vi "TempMonitor_VoltageToTemp.vi"(1 "Output Voltage":dbl) -> (0 "Temp (C)":dbl)   [LabVIEW 2012]
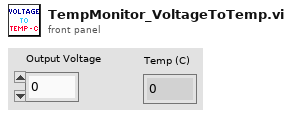
[diagram p1: front panel]
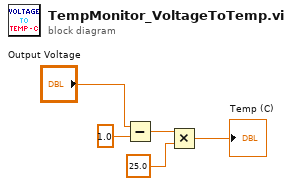
[diagram p0: block diagram]
diagram:
  n1 = Subtract(x="Output Voltage", y=1.0) -> (x-y=w4:dbl)
  n2 = Multiply(x=w4, y=25.0) -> (x*y=→"Temp (C)":dbl)
